vi "Items Mouse Click.vi"(6 "PlatMods":T1, 7 "Mods":cluster{"Double Click":bool, "Menu Key":bool}, 8 "error in (no error)":errorcluster, 9 "Button":u16, 10 "Coords":T2, 11 "Sequence Controller in":refnum<class "Sequence Controller.lvclass">) -> (0 "error out":errorcluster, 1 "Valid":bool, 2 "Name":string, 3 "Sequence Controller out":refnum<class "Sequence Controller.lvclass">, 4 "Double click":bool, 5 "In symbol":bool)   [LabVIEW 2018, in "Sequence Controller.lvclass"]
uses:
  Sequence Controller.lvclass
  C:/Program Files/National Instruments/LabVIEW 2018/vi.lib/ActorFramework/Actor/Actor.lvclass
  C:/github/LabActor/Template Module/Template Module.lvclass
  <vilib>/Utility/miscctls.llb/LVPoint32TypeDef.ctl
  <vilib>/ActorFramework/Actor/Actor.lvclass/Actor.ctl
  Template Module/Template Module.lvclass/Template Module.ctl
  Application Controller Messages/Launch Object by Type Msg/Launch Object by Type Msg.lvclass/Launch Object by Type Msg.ctl
  <vilib>/ActorFramework/Message Enqueuer/Message Enqueuer.lvclass/Message Enqueuer.ctl
  Template Module/Read Name.vi
  <vilib>/ActorFramework/Message Enqueuer/Enqueue.vi
  Application Controller Messages/Launch Object by Type Msg/Launch Object by Type Msg.lvclass
  C:/Program Files/National Instruments/LabVIEW 2018/vi.lib/ActorFramework/Message/Message.lvclass
  <vilib>/ActorFramework/Message Priority Queue/Priority Enqueue.vi
  Process Controller/Process Controller.lvclass
  <vilib>/ActorFramework/Actor/Actor.lvclass
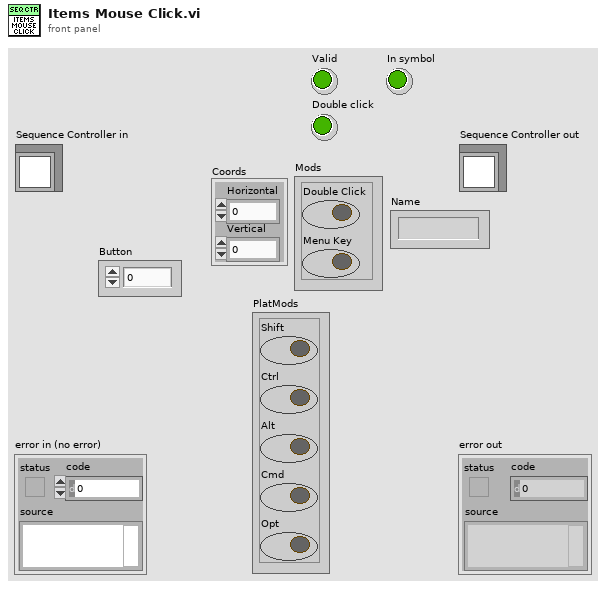
[diagram p1: front panel]
types:
  T1 = cluster{"Shift":bool, "Ctrl":bool, "Alt":bool, "Cmd":bool, "Opt":bool}
  T2 = typedef "LVPoint32TypeDef.ctl" = cluster{"Horizontal":i32, "Vertical":i32}
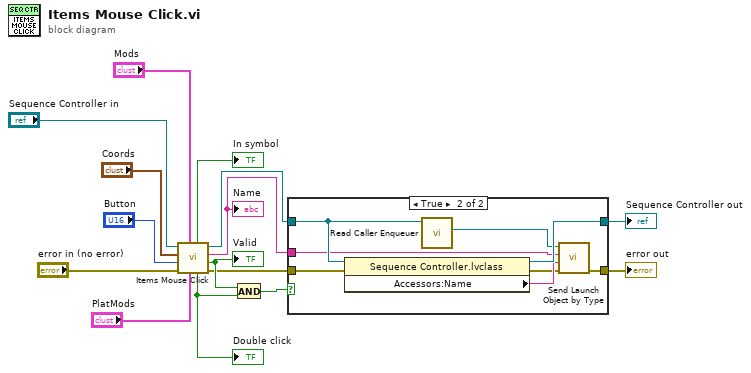
[diagram p0: block diagram]
diagram:
  n1 = call-parent "Items Mouse Click.vi"("PlatMods"="PlatMods", "Mods"="Mods", "error in (no error)"="error in (no error)", "Button"="Button", "Coords"="Coords", "Sequence Element in"="Sequence Controller in") -> ("error out"=w5:errorcluster, "Valid"=w9:bool, "Name"=w6:string, "Sequence Element out"=w3:refnum<class "Sequence Controller.lvclass">, "Double click"=w8:bool, "In symbol"=→"In symbol":bool)
  "Valid" <- w9
  "Double click" <- w8
  "Name" <- w6
  n2 = And(x=w9, y=w8) -> (x .and. y?=w7:bool)
  n3 = case shown="True" w7 {
    tunnel: w3 -> [w17 w23]
    tunnel: w6 -> [_ w21]
    tunnel: w5 -> [w16 w25]
    tunnel: [w16 w18] -> w4
    tunnel: [w17 w24] -> w2
    frame False {
    }
    frame True {
      n4 = property class="Sequence Controller.lvclass"(reference=w23, error in=w25) -> (reference out=w24:refnum<class "Sequence Controller.lvclass">, error out=w19:errorcluster, "Accessors:Name"=w22:string)
      n5 = call <vilib>:"Read Caller Enqueuer.vi"("Actor"=w23) -> ("Caller Enqueuer"=w20:refnum<class "Message Enqueuer.lvclass">)  [unwired: 10 in]
      n6 = call "Send Launch Object by Type.vi"("error in (no error)"=w19, "Requestor"=w22, "Type"=w21, "Message Enqueuer"=w20) -> ("error out"=w18:errorcluster)  [unwired: 6 in, 1 out]
    }
  }
  "error out" <- w4
  "Sequence Controller out" <- w2
